vi "Write Digital.vi"(8 "error in":errorcluster, 10 "Digital":bool[](array[boolean]), 11 "DIG_IO in":refnum<class "DIG_IO.lvclass">) -> (0 "error out":errorcluster, 3 "DIG_IO out":refnum<class "DIG_IO.lvclass">)   [LabVIEW 2019, in "DIG_IO.lvlib" / "DIG_IO.lvclass"]
uses:
  Library/DIG_IO.lvclass
  Library/DIG_IO.lvclass/DIG_IO.ctl
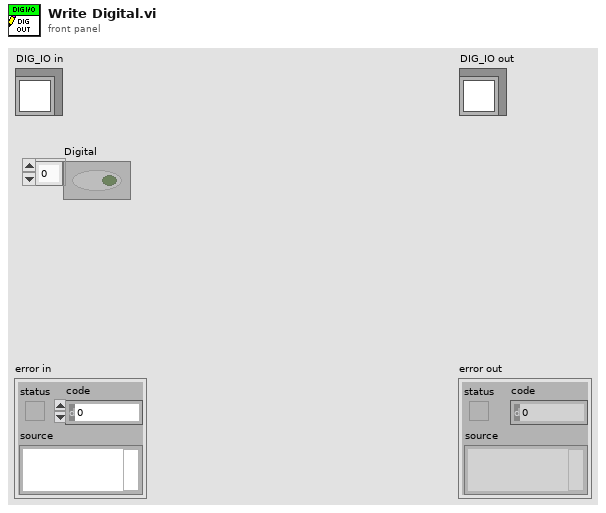
[diagram p1: front panel]
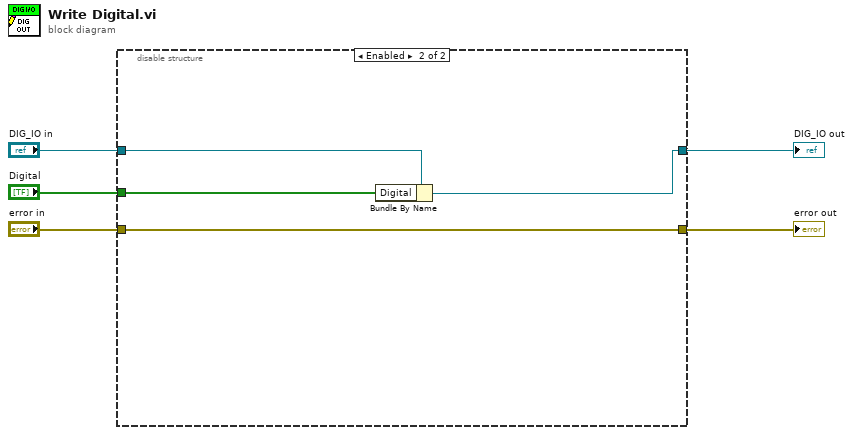
[diagram p0: block diagram]
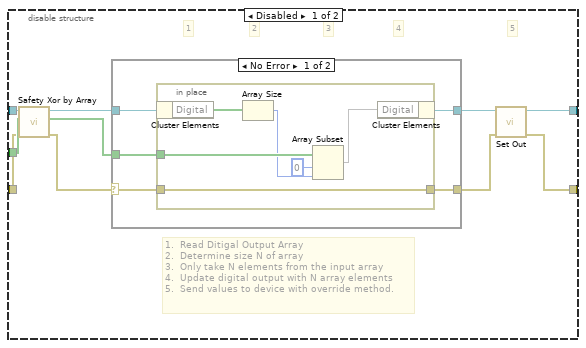
[diagram p2: hidden frame]
diagram:
  n1 = disable-structure shown="Enabled" {
    disable-tunnel: [w14 w30] -> w5
    disable-tunnel: [w12 w29] -> w4
    disable-tunnel: "DIG_IO in" -> [w11 w32]
    disable-tunnel: "Digital" -> [w9 w31]
    disable-tunnel: "error in" -> [w7 w29]
    frame Disabled {
      # "4"
      # "3"
      # "2"
      # "1.  Read Ditigal Output Array\n2.  Determine size N of array\n3.  Only take N elements from the input array\n4.  Update digital output with N array elements\n5.  Send values to device with override method."
      # "5"
      # "1"
      n2 = call "Safety Xor by Array.vi"("error in (no error)"=w7, "Digital In"=w9, "DIG_IO in"=w11) -> ("error out"=w6:errorcluster, "Digital Out"=w8:bool[], "DIG_IO out"=w10:refnum<class "DIG_IO.lvclass">)  [unwired: 6 in]
      n3 = case shown="No Error" w6 {
        selector: w6 -> [w17 w27]
        tunnel: [w16 w27] -> w13
        tunnel: [w18 w28] -> w15
        tunnel: w10 -> [w20 w28]
        tunnel: w8 -> [w19 _]
        frame No Error {
          n4 = in-place {
            in-place-border: w19 -> [w25]
            in-place-border: w17 -> [w21]
            in-place-border: [w21] -> w16
            n5 = in-place-cluster #1(w20) -> ("Digital"=w26:bool[])
            n6 = Array Size(array=w26) -> (size(s)=w24:i32)
            n7 = Array Subset(array=w25, index=0, length=w24) -> (w22:bool[])
            n8 = in-place-cluster #1("Digital"=w22) -> (w18:refnum<class "DIG_IO.lvclass">)
          }
        }
        frame Error {
        }
      }
      n9 = call-dynamic "Set Out.vi"("error in"=w13, "DIG_IO in"=w15) -> ("error out"=w12:errorcluster, "DIG_IO out"=w14:refnum<class "DIG_IO.lvclass">)  [unwired: 8 in]
    }
    frame Enabled {
      n10 = Bundle By Name(cluster=w32, "Digital"=w31) -> (w30:refnum<class "DIG_IO.lvclass">)
    }
  }
  "error out" <- w4
  "DIG_IO out" <- w5
